vi "Refresh MCL (action).vi"(8 "Error In":errorcluster, 9 "Display Order":T1, 10 "Errors To Display":T2[](array[typedef]), 11 "MCL Reference":refnum<vi>) -> (0 "Error Out":errorcluster)   [LabVIEW 2023, in "Error Manager.lvlib" / "MCL.lvclass"]
doc: "Blank VI with error handling."
uses:
  Private VIs/Handled Error (cluster).ctl
  Private VIs/Read-Unread Status (enum).ctl
  Private VIs/Display Order (enum).ctl
  MCL.lvclass
  MCL.lvclass/MCL.ctl
  Error Manager.lvlib
panel:
  # "Input\nInputs to the VI"
  # "Development\nControls or indicators that are useful for development or testing, but which are not outputs of the VI."
  # "Output\nOutputs of the VI"
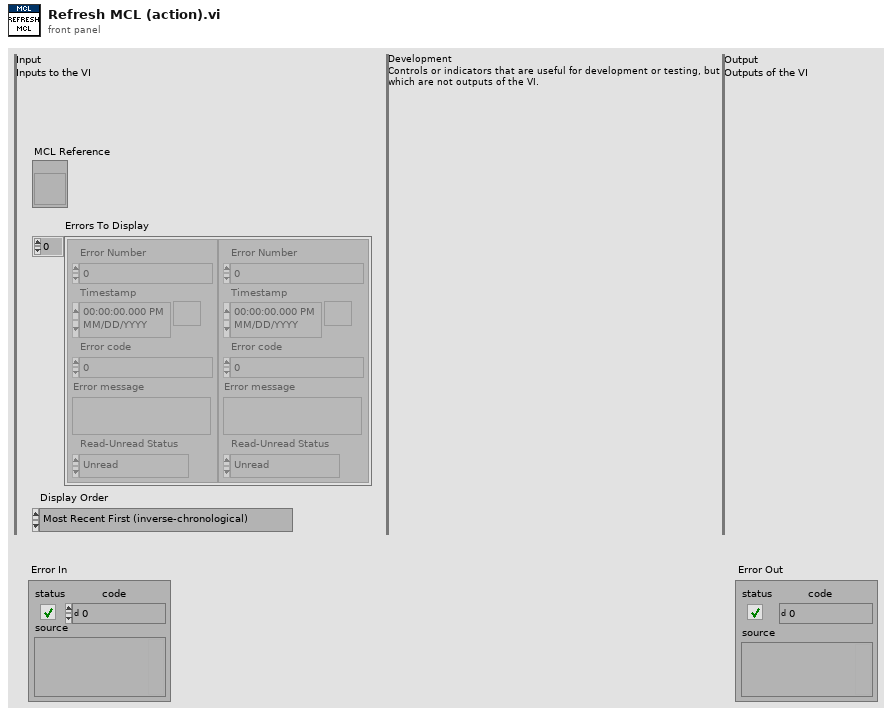
[diagram p1: front panel]
types:
  T1 = typedef "Error Manager.lvlib/Display Order (enum).ctl" = enum16{"Most Recent First (inverse-chronological)", "Oldest First (chronological)"}
  T2 = typedef "Error Manager.lvlib/Handled Error (cluster).ctl" = cluster{"Error Number":i32, "Timestamp":timestamp, "Error code":i32, "Error message":string, "Read-Unread Status":T3}
  T3 = typedef "Error Manager.lvlib/Read-Unread Status (enum).ctl" = enum16{"Unread", "Read"}
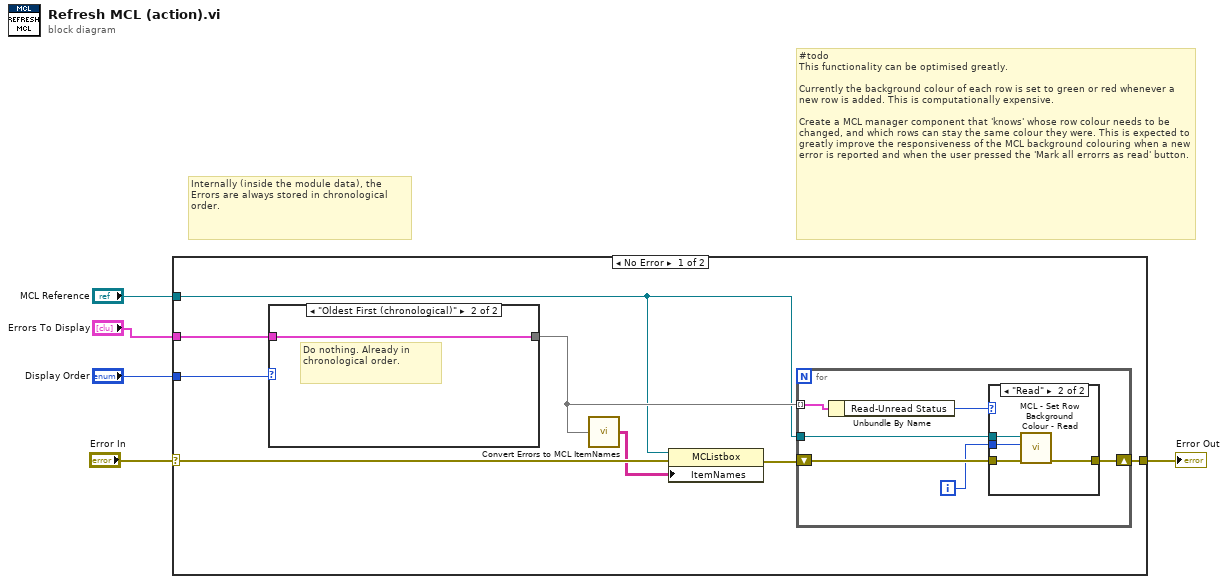
[diagram p0: block diagram]
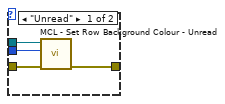
[diagram p2: hidden frame]
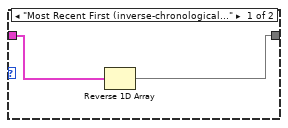
[diagram p3: hidden frame]
diagram:
  # "Internally (inside the module data), the Errors are always stored in chronological order."
  # "#todo\nThis functionality can be optimised greatly.\n\nCurrently the background colour of each row is set to green or red whenever a new row is added. This is computationally expensive.\n\nCreate a MCL manager component that 'knows' whose row colour needs to be changed, and which rows can stay the same colour they were. This is expected to greatly improve the responsiveness of the MCL background colouring when a new error is reported and when the user pressed the 'Mark all errorrs as read' button."
  n1 = case shown="No Error" "Error In" {
    selector: "Error In" -> [w13 w31]
    tunnel: [w12 w31] -> w4
    tunnel: "MCL Reference" -> [w7 _]
    tunnel: "Errors To Display" -> [w11 _]
    tunnel: "Display Order" -> [w9 _]
    frame No Error {
      n2 = case shown="\"Oldest First (chronological)\"" w9 {
        tunnel: w11 -> [w29 w30]
        tunnel: [w28 w30] -> w10
        frame "Most Recent First (inverse-chronological)" {
          n3 = Reverse 1D Array(array=w29) -> (reversed array=w28:T2[])
        }
        frame "Oldest First (chronological)" {
          # "Do nothing. Already in chronological order."
        }
      }
      n4 = call "Convert Errors to MCL ItemNames.vi"("Errors To Display"=w10) -> ("ItemNames"=w6:string[][])
      n5 = property class="MCListbox"(reference=w7, error in=w13, "ItemNames"=w6) -> (error out=w8:errorcluster)  [unwired: 1 out]
      n6 = for {
        shift-right: [w18] -> w12
        shift-left: w8 -> [w19]
        tunnel: w10 -> [w17] mode=indexing
        tunnel: w7 -> [w15]
        i -> [w14]
        n7 = Unbundle By Name(w17) -> ("Read-Unread Status"=w16:T3)
        n8 = case shown="\"Read\"" w16 {
          tunnel: w19 -> [w23 w27]
          tunnel: [w22 w26] -> w18
          tunnel: w15 -> [w21 w25]
          tunnel: w14 -> [w20 w24]
          frame "Unread" {
            n9 = call "MCL - Set Row Background Colour - Unread.vi"("error in (no error)"=w23, "Row index"=w20, "MCL Reference"=w21) -> ("error out"=w22:errorcluster)  [unwired: 8 in]
          }
          frame "Read" {
            n10 = call "MCL - Set Row Background Colour - Read.vi"("error in (no error)"=w27, "Row index"=w24, "MCL"=w25) -> ("error out"=w26:errorcluster)  [unwired: 8 in]
          }
        }
      }
    }
    frame Error {
    }
  }
  "Error Out" <- w4
